vi "LIA Simulation White Paper Host.vi"() -> ()   [LabVIEW 2017]
uses:
  <vilib>/rvi/FXPMathLib/FxpSinAndCos/subVIs/nifxpmath_SinAndCos_SimConfig.ctl
  <instrlib>/_niInstr/DSP/v1/Shared/Public/IQ Data.ctl
  <vilib>/rvi/FXPMathLib/FxpSinAndCos/simVIs/DllFxpSinAndCosTemp_sub.vi
  <vilib>/measure/maspectr.llb/FFT Power Spectrum and PSD for 1 Chan (CDB).vi
  <vilib>/rvi/FXPMathLib/FxpAdd/XNode/nifxpmath_Add.xnode
  <vilib>/rvi/FXPMathLib/FxpSinAndCos/XNode/nifxpmath_SinAndCos.xnode
  <vilib>/rvi/FXPMathLib/sim/FxpSim.dll
  <vilib>/rvi/FXPMathLib/FxpMul/XNode/nifxpmath_Multiplier.xnode
  <vilib>/rvi/FXPMathLib/FxpSub/XNode/nifxpmath_Sub.xnode
  <vilib>/ptbypt/NI_PtbyPt.lvlib
  <vilib>/measure/NI_MAPro.lvlib
  <instrlib>/_niInstr/DSP/v1/FPGA/niInstr DSP v1 FPGA.lvlib
  <instrlib>/_niInstr/DSP/v1/Shared/niInstr DSP v1 Shared.lvlib
  <vilib>/Analysis/NI_AALBase.lvlib
panel:
  out "Std Dev":dbl=1000000.0 format="%#_p"
  out "Mean":dbl=1000000.0 format="%#_p"
  out "phase delta (pi rad) 2":fxp<+/-,32,1>
  out "Waveform Graph 2":cluster{"f0":dbl, "df":dbl, "magnitude":dbl[]}[](graph)
  in  "Frequency (Hz)":dbl=1000000.0 format="%#_p"
  in  "Sampling Rate (Hz)":dbl=100000000.0 format="%#_p"
  out "Waveform Graph":dbl[][](graph)
  out "phase delta (pi rad) 1":fxp<+/-,25,1>
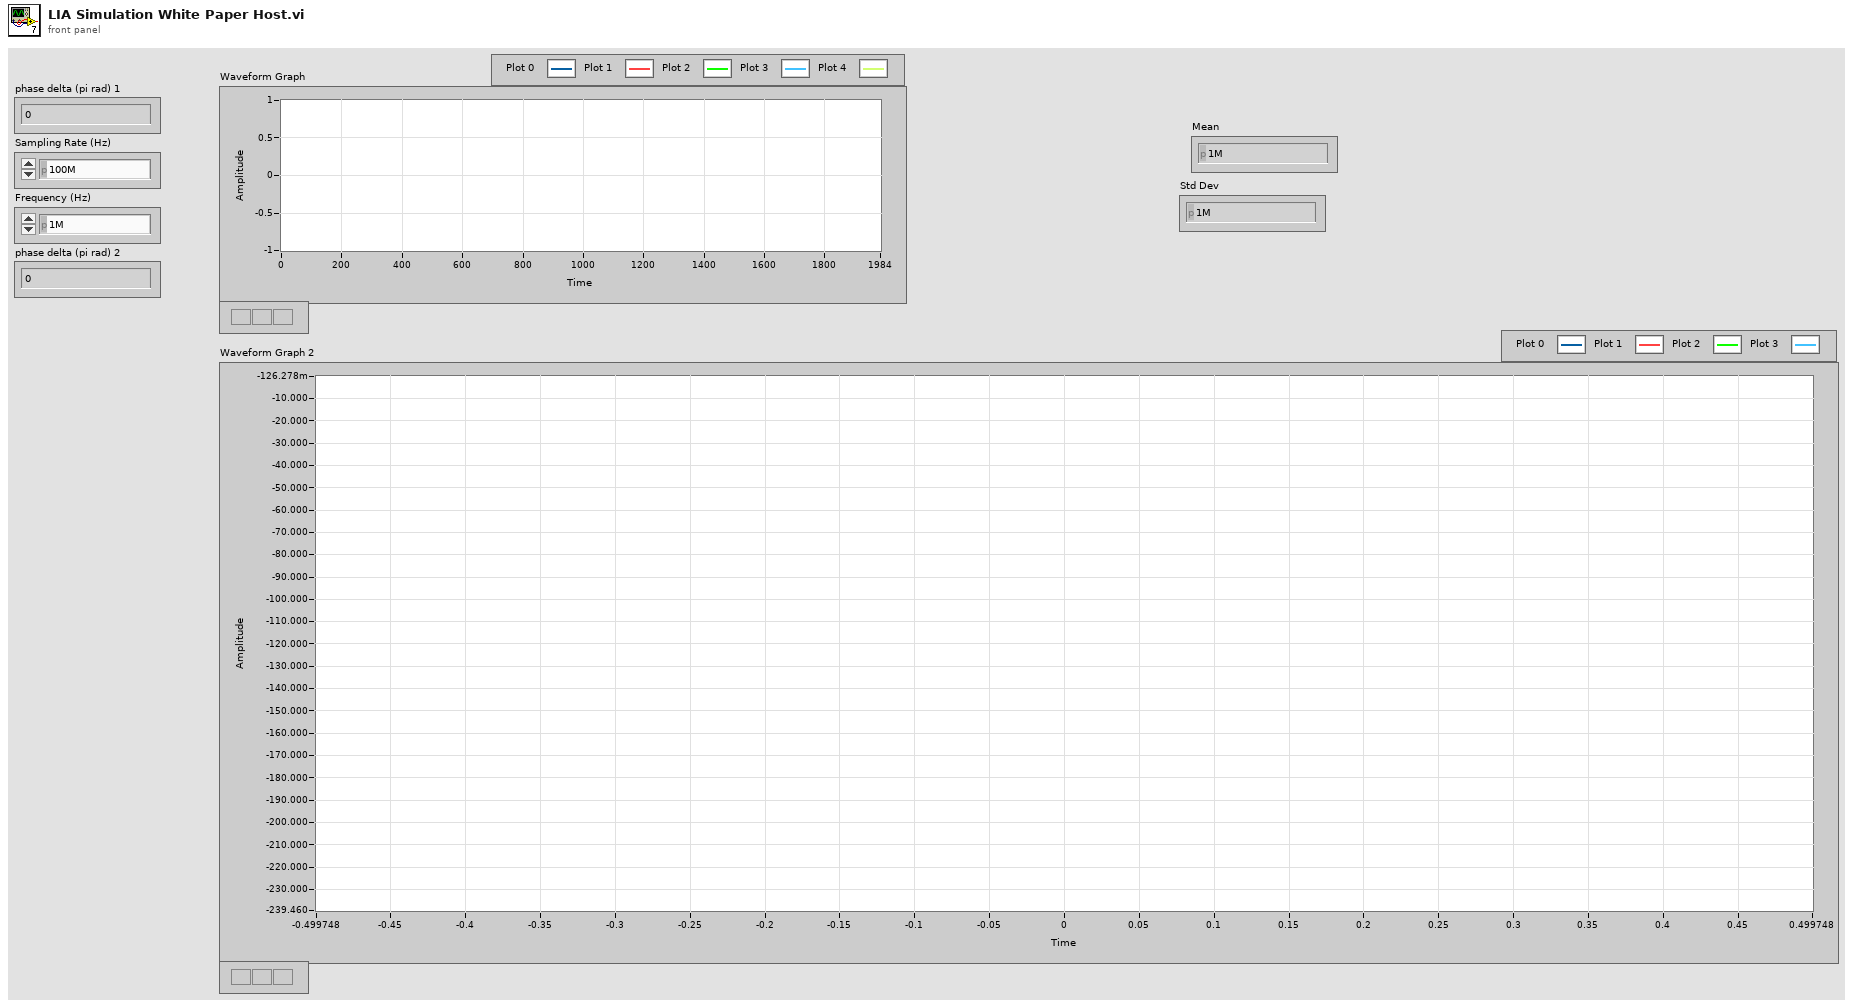
[diagram p1: front panel]
types:
  T1 = typedef "niInstr DSP v1 Shared.lvlib/IQ Data.ctl" = cluster{"I":fxp<+/-,18,1>, "Q":fxp<+/-,18,1>, "overflow":bool}
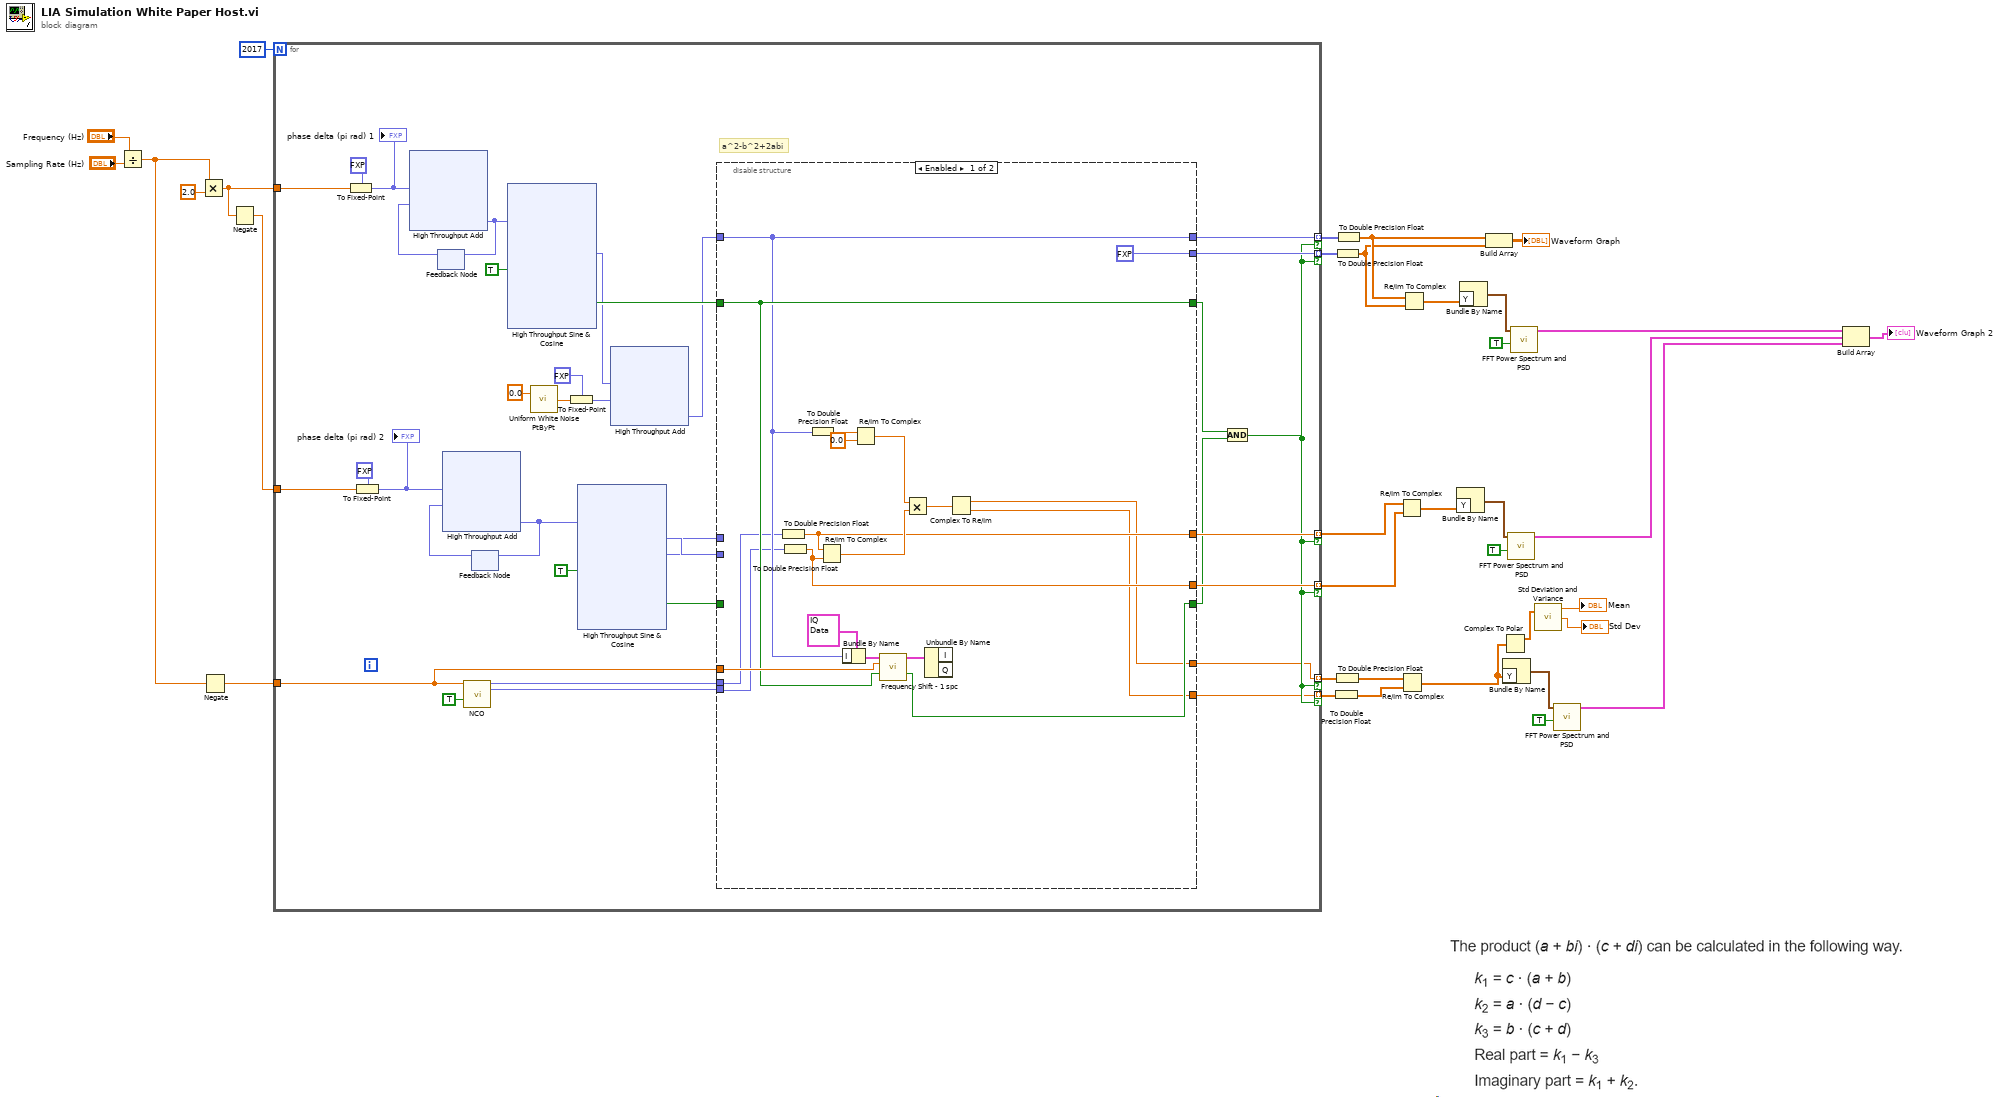
[diagram p0: block diagram]
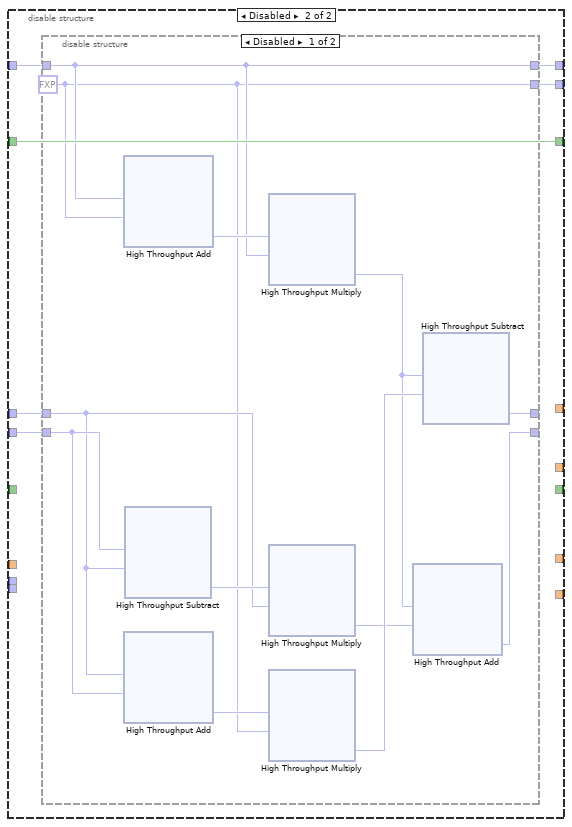
[diagram p2: hidden frame]
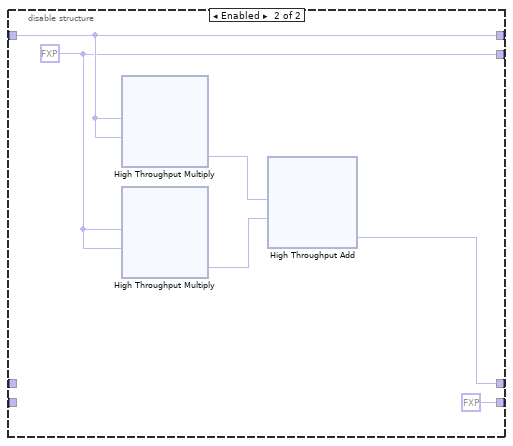
[diagram p3: hidden frame]
diagram:
  n1 = Divide(x="Frequency (Hz)", y="Sampling Rate (Hz)") -> (x/y=w21:dbl)
  n2 = Multiply(x=w21, y=2.0) -> (x*y=w25:dbl)
  n3 = Negate(x=w21) -> (-x=w20:dbl)
  n4 = Negate(x=w25) -> (-x=w24:dbl)
  n5 = for {
    N: 2017 -> [_]
    tunnel: [w57] -> w31 mode=indexing if=w39
    tunnel: w25 -> [w69]
    tunnel: [w56] -> w30 mode=indexing if=w39
    tunnel: w24 -> [w60]
    tunnel: [w38] -> w2 mode=indexing if=w39
    tunnel: [w37] -> w1 mode=indexing if=w39
    tunnel: w20 -> [w46]
    tunnel: [w41] -> w10 mode=indexing if=w39
    tunnel: [w40] -> w7 mode=indexing if=w39
    # "a^2-b^2+2abi"
    n6 = To Fixed-Point(fixed-point type=fxp<+/-,25,1> 0.0, number=w69) -> (fixed-point=w68:fxp<+/-,25,1>)
    "phase delta (pi rad) 1" <- w68
    n7 = To Fixed-Point(fixed-point type=fxp<+/-,32,1> 0.0 ("phase delta (pi rad)"), number=w60) -> (fixed-point=w63:fxp<+/-,32,1>)
    "phase delta (pi rad) 2" <- w63
    n8 = feedback #1() -> (w66:fxp<+/-,25,2>)  [unwired: 1 in]
    n9 = xnode ("High Throughput Add")("x"=w68, "y"=w66) -> ("x+y"=w70:fxp<+/-,25,2>)
    n10 = feedback-in #1(w70) -> ()
    n11 = call <instrlib>:"NCO.vi"("frequency"=w46, "input valid"=TRUE) -> ("cosine out"=w49:fxp<+/-,18,1>, "sine out"=w48:fxp<+/-,18,1>)  [unwired: 11 in, 1 out]
    n12 = feedback #2() -> (w65:fxp<+/-,32,2>)  [unwired: 1 in]
    n13 = xnode ("High Throughput Add")("x"=w63, "y"=w65) -> ("x+y"=w61:fxp<+/-,32,2>)
    n14 = feedback-in #2(w61) -> ()
    n15 = xnode "High Throughput Sine & Cosine"("x (pi)"=w70, "input valid"=TRUE) -> ("cos(x)"=w53:fxp<+/-,16,2>, "output valid"=w55:bool)  [unwired: 1 in, 2 out]
    n16 = call <vilib>:"Uniform White Noise PtByPt.vi"("amplitude"=0.0) -> ("uniform white noise"=w51:dbl)  [unwired: 2 in]
    n17 = To Fixed-Point(fixed-point type=fxp<+/-,18,1> 0.0, number=w51) -> (fixed-point=w45:fxp<+/-,18,1>)
    n18 = xnode "High Throughput Sine & Cosine"("x (pi)"=w61, "input valid"=TRUE) -> ("sin(x)"=w59:fxp<+/-,32,2>, "cos(x)"=w58:fxp<+/-,32,2>, "output valid"=w42:bool)  [unwired: 1 in, 1 out]
    n19 = xnode ("High Throughput Add")("x"=w53, "y"=w45) -> ("x+y"=w44:fxp<+/-,16,2>)
    n20 = disable-structure shown="Enabled" {
      disable-tunnel: w59 -> [_ w93]
      disable-tunnel: w58 -> [_ w92]
      disable-tunnel: [w82 w91] -> w57
      disable-tunnel: [fxp<+/-,25,2> 0.0 ("x+y") w90] -> w56
      disable-tunnel: w44 -> [w82 w94]
      disable-tunnel: [w84 w96] -> w36
      disable-tunnel: [w83 w95] -> w43
      disable-tunnel: w55 -> [w83 w95]
      disable-tunnel: w49 -> [w74 _]
      disable-tunnel: w48 -> [w73 _]
      disable-tunnel: w46 -> [w86 _]
      disable-tunnel: w42 -> [_ _]
      disable-tunnel: [w76 _] -> w41
      disable-tunnel: [w75 _] -> w40
      disable-tunnel: [w72 _] -> w38
      disable-tunnel: [w71 _] -> w37
      frame Enabled {
        n21 = To Double Precision Float(number=w74) -> (double precision float=w76:dbl)
        n22 = To Double Precision Float(number=w73) -> (double precision float=w75:dbl)
        n23 = To Double Precision Float(number=w82) -> (double precision float=w81:dbl)
        n24 = Re/Im To Complex(1:w75, 2:w76) -> (0:w78:cdb)
        n25 = Bundle By Name(cluster=T1 {"I"=0.0, "Q"=0.0, "overflow"=FALSE} ("data in"), "I"=w82) -> (w87:T1)
        n26 = Re/Im To Complex(1:0.0 ("y"), 2:w81) -> (0:w79:cdb)
        n27 = call <instrlib>:"Frequency Shift - 1 spc.vi"("data in"=w87, "frequency shift"=w86, "input valid"=w83) -> ("data out"=w85:T1, "output valid"=w84:bool)  [unwired: 10 in, 1 out]
        n28 = Multiply(x=w79, y=w78) -> (x*y=w77:cdb)
        n29 = Unbundle By Name(w85) -> ()  [unwired: 2 out]
        n30 = Complex To Re/Im(x + iy=w77) -> (x=w72:dbl, y=w71:dbl)
      }
      frame Disabled {
        n31 = disable-structure shown="Disabled" {
          disable-tunnel: w94 -> [w98 w112]
          disable-tunnel: [w104 w110] -> _
          disable-tunnel: [w101 fxp<+/-,21,3> 0.0 ("x-y")] -> _
          disable-tunnel: w93 -> [w100 _]
          disable-tunnel: w92 -> [w99 _]
          disable-tunnel: [w98 w112] -> w91
          disable-tunnel: [w97 w109] -> w90
          frame Disabled {
            w97 = fxp<+/-,25,2> 0.0 ("y")
            n32 = xnode ("High Throughput Add")("x"=w98, "y"=w97) -> ("x+y"=w108:fxp<+/-,22,2>)
            n33 = xnode ("High Throughput Add")("x"=w99, "y"=w100) -> ("x+y"=w106:fxp<+/-,22,2>)
            n34 = xnode ("High Throughput Subtract")("x"=w100, "y"=w99) -> ("x-y"=w107:fxp<+/-,33,3>)
            n35 = xnode ("High Throughput Multiply")("x"=w108, "y"=w98) -> ("x*y"=w103:fxp<+/-,20,2>)
            n36 = xnode ("High Throughput Multiply")("x"=w107, "y"=w99) -> ("x*y"=w102:fxp<+/-,20,2>)
            n37 = xnode ("High Throughput Multiply")("x"=w106, "y"=w97) -> ("x*y"=w105:fxp<+/-,20,2>)
            n38 = xnode ("High Throughput Add")("x"=w103, "y"=w102) -> ("x+y"=w101:fxp<+/-,22,2>)
            n39 = xnode ("High Throughput Subtract")("x"=w103, "y"=w105) -> ("x-y"=w104:fxp<+/-,21,3>)
          }
          frame Enabled {
            w109 = fxp<+/-,25,2> 0.0 ("x")
            n40 = xnode ("High Throughput Multiply")("x"=w112, "y"=w112) -> ("x*y"=w114:fxp<+/-,25,2>)
            n41 = xnode ("High Throughput Multiply")("x"=w109, "y"=w109) -> ("x*y"=w113:fxp<+/-,25,2>)
            n42 = xnode ("High Throughput Add")("x"=w114, "y"=w113) -> ("x+y"=w110:fxp<+/-,25,2>)
          }
        }
      }
    }
    n43 = And(x=w43, y=w36) -> (x .and. y?=w39:bool)
  }
  n44 = To Double Precision Float(number=w1) -> (double precision float=w23:dbl[])
  n45 = To Double Precision Float(number=w2) -> (double precision float=w22:dbl[])
  n46 = To Double Precision Float(number=w30) -> (double precision float=w28:dbl[])
  n47 = To Double Precision Float(number=w31) -> (double precision float=w29:dbl[])
  n48 = Re/Im To Complex(1:w7, 2:w10) -> (0:w11:cdb[])
  n49 = Re/Im To Complex(1:w23, 2:w22) -> (0:w6:cdb[])
  n50 = Re/Im To Complex(1:w28, 2:w29) -> (0:w19:cdb[])
  n51 = Bundle By Name("Y"=w11) -> (w12:waveform(cdb))  [unwired: 1 in]
  n52 = Bundle By Name("Y"=w19) -> (w18:waveform(cdb))  [unwired: 1 in]
  n53 = Build Array(w29, w28) -> (→"Waveform Graph":dbl[][])
  n54 = Complex To Polar(r * e^(i*theta)=w6) -> (r=w5:dbl[])  [unwired: 1 out]
  n55 = Bundle By Name("Y"=w6) -> (w16:waveform(cdb))  [unwired: 1 in]
  n56 = call-poly <vilib>:"FFT Power Spectrum and PSD.vi"("dB On (F)"=TRUE, "time signal"=w12) -> ("Power Spectrum / PSD"=w9:cluster{"f0":dbl, "df":dbl, "magnitude":dbl[]})  [unwired: 6 in, 3 out]
  n57 = call-poly <vilib>:"FFT Power Spectrum and PSD.vi"("dB On (F)"=TRUE, "time signal"=w18) -> ("Power Spectrum / PSD"=w14:cluster{"f0":dbl, "df":dbl, "magnitude":dbl[]})  [unwired: 6 in, 3 out]
  n58 = call <vilib>:"Std Deviation and Variance.vi"("X"=w5) -> ("mean"=→"Mean":dbl, "standard deviation"=→"Std Dev":dbl)  [unwired: 1 in, 1 out]
  n59 = call-poly <vilib>:"FFT Power Spectrum and PSD.vi"("dB On (F)"=TRUE, "time signal"=w16) -> ("Power Spectrum / PSD"=w8:cluster{"f0":dbl, "df":dbl, "magnitude":dbl[]})  [unwired: 6 in, 3 out]
  n60 = Build Array(w14, w9, w8) -> (→"Waveform Graph 2":cluster{"f0":dbl, "df":dbl, "magnitude":dbl[]}[])
